vi "svc_Check for Resampled Signal Continuity (N Ch).vi"(0 "even angle signals":T5(array[cluster]) {"even angle signal" format="%.2f"; "dr" format="%.2f"; "r0" format="%.2f"}, 1 "restart averaging (F)":bool, 5 "even angle channel info":T1[](array[typedef]) {"channel info"."pregain" format="%.2f"; "channel info"."weighting filter" items=["Linear", "A-weighting", "B-weighting", "C-weighting", "ITU-R 468-4", "Dolby", "CCITT", "C-message", "Wb", "Wc", "Wd", "We", "Wf", "Wh", "Wj", "Wk", "Wm", "AES17 20 kHz lowpass", "AES17 40 kHz lowpass", "AES17 20 kHz highpass", "AES17 40 kHz highpass"]; "channel info"."dB reference" format="%^.1e"; "channel info"."engineering units" items=["custom..."=0, "V"=1, "A"=21, "C"=30, "pC"=31, "s"=32, "-"=29, "Pa"=2, "N"=20, "g"=3, "m/s^2"=4, "m/s"=5, "m"=6, "mm/s"=12, "mm"=13, "micron/s"=14, "micron"=15, "in/s^2"=7, "in/s"=8, "in"=9, "mil/s"=10, "mil"=11, "rad/s^2"=16, "rad/s"=17, "rad"=18, "deg/s^2"=26, "deg/s"=27, "deg"=28, "RPM"=22, "cycle/s^2"=23, "Hz"=24, "cycle"=25, "strain"=19]; "channel info"."sensor sensitivity" format="%#_5f"}, 7 "parameter controls":T7, 9 "multichannel parameter controls":T6, 11 "error in (no error)":errorcluster) -> (3 "dr":dbl, 4 "dup even angle signals":T5(array[cluster]) {"even angle signal" format="%.2f"; "dr" format="%.2f"; "r0" format="%.2f"}, 6 "dup even angle channel info":T1[](array[typedef]) {"channel info"."pregain" format="%.2f"; "channel info"."weighting filter" items=["Linear", "A-weighting", "B-weighting", "C-weighting", "ITU-R 468-4", "Dolby", "CCITT", "C-message", "Wb", "Wc", "Wd", "We", "Wf", "Wh", "Wj", "Wk", "Wm", "AES17 20 kHz lowpass", "AES17 40 kHz lowpass", "AES17 20 kHz highpass", "AES17 40 kHz highpass"]; "channel info"."dB reference" format="%^.1e"; "channel info"."engineering units" items=["custom..."=0, "V"=1, "A"=21, "C"=30, "pC"=31, "s"=32, "-"=29, "Pa"=2, "N"=20, "g"=3, "m/s^2"=4, "m/s"=5, "m"=6, "mm/s"=12, "mm"=13, "micron/s"=14, "micron"=15, "in/s^2"=7, "in/s"=8, "in"=9, "mil/s"=10, "mil"=11, "rad/s^2"=16, "rad/s"=17, "rad"=18, "deg/s^2"=26, "deg/s"=27, "deg"=28, "RPM"=22, "cycle/s^2"=23, "Hz"=24, "cycle"=25, "strain"=19]; "channel info"."sensor sensitivity" format="%#_5f"}, 8 "waveform parameter changed":bool, 10 "multichannel parameter changed":bool, 14 "array length":i32, 15 "error out":errorcluster)   [LabVIEW 2017]
uses:
  <vilib>/addons/_NISVFA/_Shared subVIs/Controls/svc_Resampled Channel Info.ctl
  <vilib>/addons/_NISVFA/_Shared subVIs/Controls/svc_Channel Info.ctl
  <vilib>/addons/_NISVFA/_Shared subVIs/Controls/svc_Engineering Units Text Ring.ctl
  <vilib>/addons/_NISVFA/_Shared subVIs/Controls/svc_Weighting Filter Text Ring.ctl
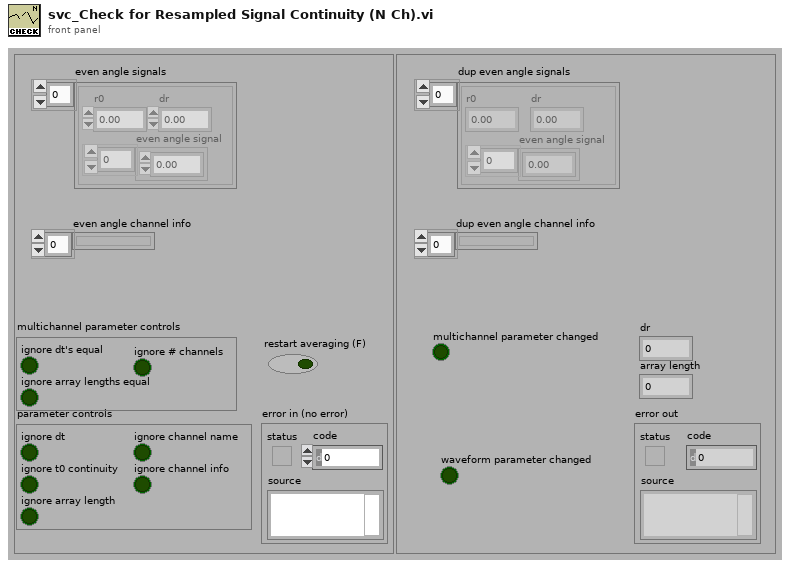
[diagram p1: front panel]
types:
  T1 = typedef "svc_Resampled Channel Info.ctl" = cluster{"channel name":string, "description":string, " channel info":T2}
  T2 = typedef "svc_Channel Info.ctl" = cluster{"sensor sensitivity":dbl, "engineering units":T3, "dB reference":dbl, "custom label":string, "weighting filter":T4, "pregain":dbl}
  T3 = typedef "svc_Engineering Units Text Ring.ctl" = u16
  T4 = typedef "svc_Weighting Filter Text Ring.ctl" = u16
  T5 = cluster{"r0":dbl, "dr":dbl, "even angle signal":dbl[]}[]
  T6 = cluster{"ignore dt's equal":bool, "ignore array lengths equal":bool, "ignore # channels ":bool}
  T7 = cluster{"ignore dt":bool, "ignore t0 continuity":bool, "ignore array length":bool, "ignore channel info":bool, "ignore channel name":bool}
  T8 = cluster{"r0":dbl, "dr":dbl, "array length":i32}[]
  T9 = cluster{"r0":dbl, "dr":dbl, "even angle signal":dbl[]}
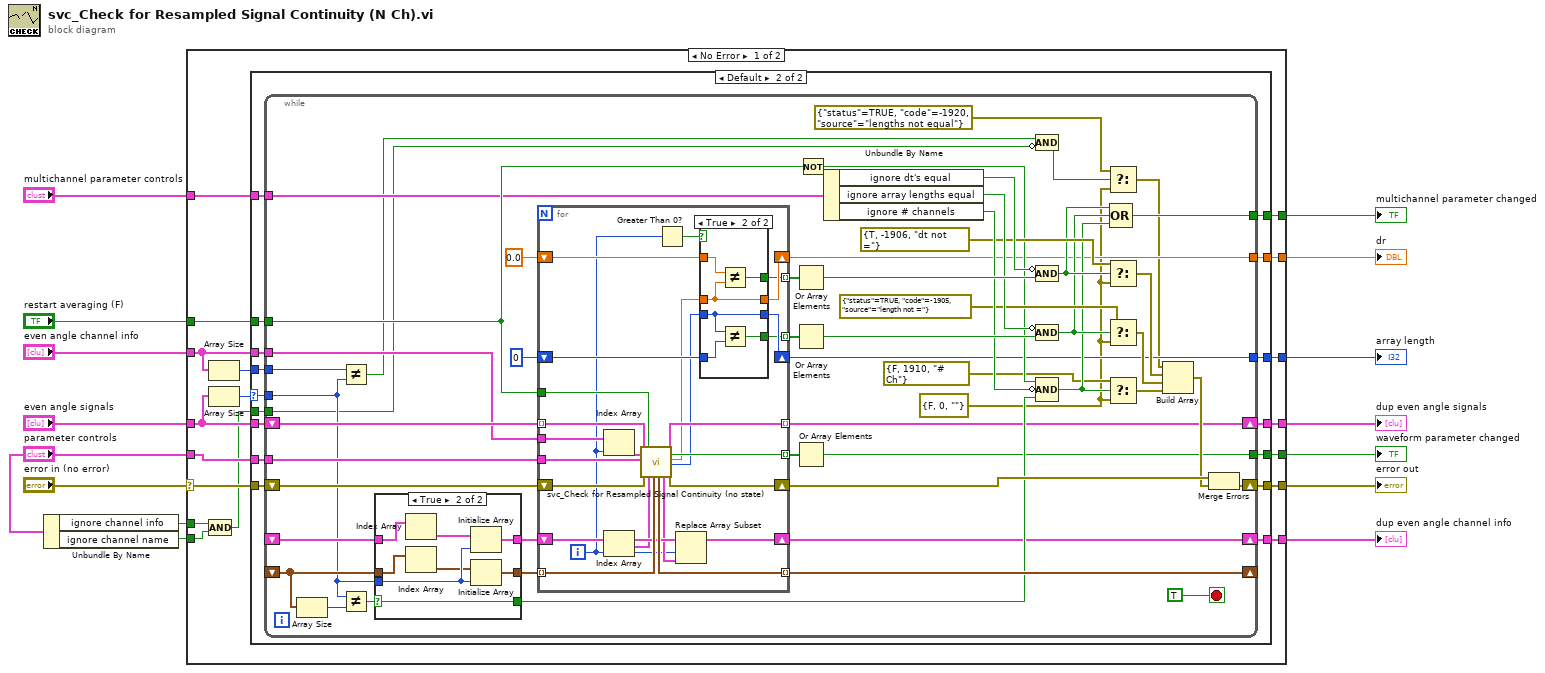
[diagram p0: block diagram]
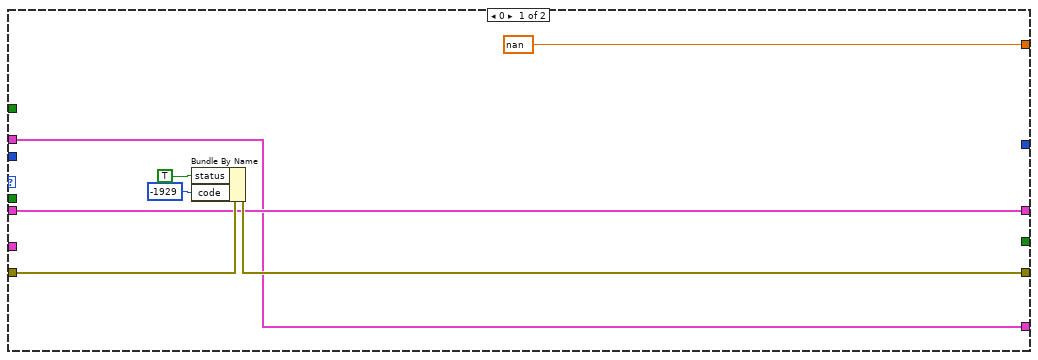
[diagram p2: hidden frame]
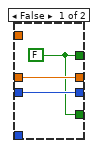
[diagram p4: hidden frame]
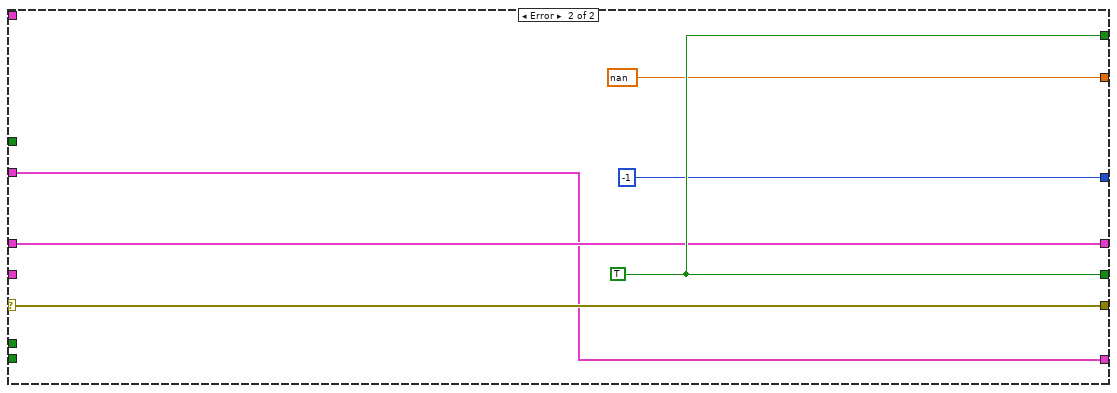
[diagram p5: hidden frame]
diagram:
  n1 = Unbundle By Name("parameter controls") -> ("ignore channel info"=w3:bool, "ignore channel name"=w2:bool)
  n2 = case shown="No Error" "error in (no error)" {
    selector: "error in (no error)" -> [w24 w159]
    tunnel: [w33 w159] -> w15
    tunnel: "parameter controls" -> [w21 _]
    tunnel: [w32 w158] -> w14
    tunnel: "even angle signals" -> [w22 w157]
    tunnel: "restart averaging (F)" -> [w31 _]
    tunnel: "multichannel parameter controls" -> [w30 _]
    tunnel: [w29 w158] -> w10
    tunnel: [w28 w157] -> w8
    tunnel: [w27 nan] -> w7
    tunnel: [w26 -1] -> w6
    tunnel: [w25 w154] -> w5
    tunnel: "even angle channel info" -> [w23 w154]
    tunnel: w3 -> [w18 _]
    tunnel: w2 -> [w17 _]
    frame No Error {
      n3 = Array Size(array=w23) -> (size(s)=w19:i32)
      n4 = Array Size(array=w22) -> (size(s)=w20:i32)
      n5 = Compound Arithmetic op=AND(w18, w17) -> (w16:bool)
      n6 = case shown="Default" w20 {
        selector: w20 -> [_ w43]
        tunnel: [w38 w56] -> w33
        tunnel: w21 -> [_ w55]
        tunnel: [_ w54] -> w32
        tunnel: w22 -> [w36 w53]
        tunnel: w31 -> [_ w52]
        tunnel: w30 -> [_ w51]
        tunnel: [_ w50] -> w29
        tunnel: [w36 w49] -> w28
        tunnel: [nan w48] -> w27
        tunnel: [_ w47] -> w26
        tunnel: [w35 w46] -> w25
        tunnel: w23 -> [w35 w45]
        tunnel: w24 -> [w39 w44]
        tunnel: w19 -> [_ w42]
        tunnel: w16 -> [_ w41]
        frame 0 {
          n7 = Bundle By Name(cluster=w39, "status"=TRUE, "code"=-1929) -> (w38:errorcluster)
        }
        frame Default {
          n8 = while {
            tunnel: w55 -> [w108]
            tunnel: [w78] -> w54
            shift-right: [w106] -> _
            shift-left: _ -> [w102]
            tunnel: w52 -> [w94]
            tunnel: w51 -> [w70]
            tunnel: [w71] -> w50
            shift-right: [w75] -> w46
            shift-left: _ -> [w74]
            shift-right: [w72] -> w49
            shift-left: w53 -> [w103]
            tunnel: [w69] -> w48
            tunnel: [w67] -> w47
            tunnel: w45 -> [w66]
            shift-right: [w97] -> w56
            shift-left: w44 -> [w65]
            tunnel: w43 -> [w62]
            tunnel: w42 -> [w61]
            tunnel: w41 -> [w58]
            stop <- TRUE stop-if-true
            w64 = errorcluster {"status"=FALSE, "code"=0, "source"=""} ("error in (no error)")
            n9 = Array Size(array=w102) -> (size(s)=w105:i32)
            n10 = Not Equal?(x=w61, y=w62) -> (x != y?=w59:bool)
            n11 = Not Equal?(x=w62, y=w105) -> (x != y?=w104:bool)
            n12 = case shown="True" w104 {
              selector: w104 -> [w110 w118]
              tunnel: w102 -> [w111 w116]
              tunnel: [w111 w119] -> w95
              tunnel: w62 -> [_ w117]
              tunnel: [w110 w118] -> w88
              tunnel: [w109 w113] -> w73
              tunnel: w74 -> [w109 w112]
              frame False {
              }
              frame True {
                n13 = Index Array(array=w112) -> (element=w114:T1)  [unwired: 1 in]
                n14 = Index Array(array=w116) -> (element=w115:cluster{"r0":dbl, "dr":dbl, "array length":i32})  [unwired: 1 in]
                n15 = Initialize Array(w114, w117) -> (w113:T1[])
                n16 = Initialize Array(w115, w117) -> (w119:T8)
              }
            }
            n17 = for {
              tunnel: w108 -> [w132]
              tunnel: w103 -> [w130] mode=indexing
              tunnel: [w144] -> w106 mode=indexing
              tunnel: w95 -> [w143] mode=indexing
              tunnel: w94 -> [w141]
              shift-right: [w142] -> w96
              shift-left: w65 -> [w131]
              tunnel: [w140] -> w76 mode=indexing
              shift-right: [w136] -> w69
              shift-left: 0.0 -> [w138]
              shift-right: [w135] -> w67
              shift-left: 0 -> [w137]
              tunnel: [w134] -> w99 mode=indexing
              tunnel: [w133] -> w98 mode=indexing
              tunnel: [w129] -> w72 mode=indexing
              shift-right: [w124] -> w75
              shift-left: w73 -> [w126]
              tunnel: w66 -> [w122]
              i -> [w121]
              n18 = Index Array(array=w122, index=w121) -> (element=w120:T1)
              n19 = Index Array(array=w126, index=w121) -> (element=w123:T1)
              n20 = call <vilib>:"svc_Check for Resampled Signal Continuity (no state).vi"("even angle signal"=w130, "even angle channel info"=w120, "parameter controls"=w132, "error in (no error)"=w131, "reset"=w141, "expected even angle channel info"=w123, "expected signal parameters"=w143) -> ("next expected signal parameters"=w144:cluster{"r0":dbl, "dr":dbl, "array length":i32}, "even angle channel info"=w125:T1, "even angle signal"=w129:T9, "waveform parameter changed"=w140:bool, "dt"=w128:dbl, "array length"=w127:i32, "error out"=w142:errorcluster)  [unwired: 6 in]
              n21 = Greater Than 0?(x=w121) -> (x > 0?=w139:bool)
              n22 = Replace Array Subset(array=w126, new element=w125, index=w121) -> (w124:T1[])
              n23 = case shown="True" w139 {
                tunnel: w128 -> [w146 w150]
                tunnel: w127 -> [w147 w151]
                tunnel: w138 -> [_ w153]
                tunnel: w137 -> [_ w152]
                tunnel: [w147 w151] -> w135
                tunnel: [w146 w150] -> w136
                tunnel: [w145 w149] -> w134
                tunnel: [w145 w148] -> w133
                frame False {
                  w145 = FALSE
                }
                frame True {
                  n24 = Not Equal?(x=w153, y=w150) -> (x != y?=w149:bool)
                  n25 = Not Equal?(x=w151, y=w152) -> (x != y?=w148:bool)
                }
              }
            }
            n26 = Or Array Elements(Boolean array=w99) -> (logical OR=w92:bool)
            n27 = Or Array Elements(Boolean array=w98) -> (logical OR=w90:bool)
            n28 = Or Array Elements(Boolean array=w76) -> (logical OR=w78:bool)
            n29 = Not(x=w94) -> (.not. x?=w77:bool)
            n30 = Unbundle By Name(w70) -> ("ignore dt's equal"=w93:bool, "ignore array lengths equal"=w91:bool, "ignore # channels"=w89:bool)
            n31 = Compound Arithmetic op=AND(w59, invert w58) -> (w60:bool)
            n32 = Compound Arithmetic op=AND(invert w93, w92) -> (w82:bool)
            n33 = Compound Arithmetic op=AND(invert w91, w90) -> (w81:bool)
            n34 = Compound Arithmetic op=AND(w77, invert w89, w88) -> (w80:bool)
            n35 = Select(t=errorcluster {"status"=TRUE, "code"=-1920, "source"="lengths not equal"} ("error in (no error)"), s=w60, f=w64) -> (s? t:f=w57:errorcluster)
            n36 = Select(t=errorcluster {"status"=TRUE, "code"=-1906, "source"="dt not ="} ("error in (no error)"), s=w82, f=w64) -> (s? t:f=w87:errorcluster)
            n37 = Select(t=errorcluster {"status"=TRUE, "code"=-1905, "source"="length not ="} ("error in (no error)"), s=w81, f=w64) -> (s? t:f=w86:errorcluster)
            n38 = Select(t=errorcluster {"status"=FALSE, "code"=1910, "source"="# Ch"} ("error in (no error)"), s=w80, f=w64) -> (s? t:f=w85:errorcluster)
            n39 = Compound Arithmetic op=OR(w82, w81, w80) -> (w71:bool)
            n40 = Build Array(w57, w87, w86, w85) -> (w79:errorcluster[])
            n41 = Merge Errors(w96, w79) -> (w97:errorcluster)
          }
        }
      }
    }
    frame Error {
      w158 = TRUE ("waveform parameter changed")
    }
  }
  "error out" <- w15
  "waveform parameter changed" <- w14
  "multichannel parameter changed" <- w10
  "dup even angle signals" <- w8
  "array length" <- w6
  "dr" <- w7
  "dup even angle channel info" <- w5
